vi "Handle Error.vi"(7 "Stop on Unhandled Error (T)":bool=TRUE, 8 "error in":errorcluster, 11 "Measurement":refnum<class "Measurement.lvclass">) -> (0 "handling error":errorcluster, 2 "Unhandled error":errorcluster, 3 "Measurement out":refnum<class "Measurement.lvclass">)   [LabVIEW 2019, in "Measurement.lvclass"]
doc: "JKI State Machine Objects (SMO) 1.0.0.11\nJKI - JKI\nCopyright (c) 2016, JKIJKI State Machine Objects (SMO) 1.3.0.56\nJKI - JKI\nCopyright (c) 2017, JKI"
uses:
  Measurement.lvclass
  <vilib>/JKI/JKI SMO/SMO/SMO.lvclass
panel:
  # "For instructions on how to use the JKI State Machine Objects, examples and video tutorials, visit:\nhttp://jki.net/state-machine-objects/\n\nJKI State Machine Objects™\nhttp://jki.net/state-machine-objects/\nCopyright (C) 2005-2015, JKI <info@jki.net>\nALL RIGHTS RESERVED"
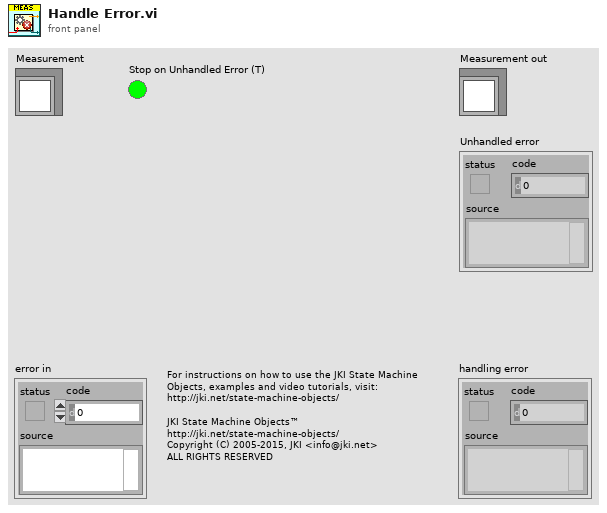
[diagram p1: front panel]
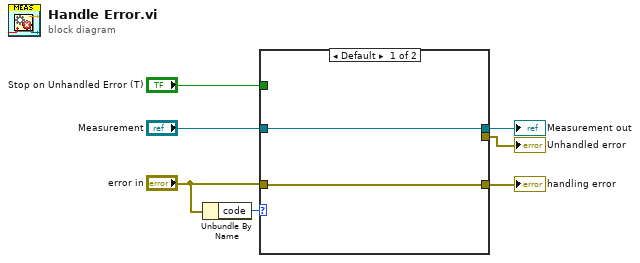
[diagram p0: block diagram]
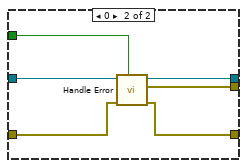
[diagram p2: hidden frame]
diagram:
  n1 = Unbundle By Name("error in") -> ("code"=w7:i32)
  n2 = case shown="Default" w7 {
    tunnel: "error in" -> [w8 w12]
    tunnel: "Measurement" -> [w9 w15]
    tunnel: [w9 w14] -> w4
    tunnel: "Stop on Unhandled Error (T)" -> [_ w13]
    tunnel: [w8 w11] -> w2
    tunnel: [_ w10] -> w1
    frame Default {
    }
    frame 0 {
      n3 = call-parent "Handle Error.vi"("Stop on Unhandled Error (T)"=w13, "error in"=w12, "SMO"=w15) -> ("handling error"=w11:errorcluster, "Unhandled error"=w10:errorcluster, "SMO out"=w14:refnum<class "Measurement.lvclass">)  [unwired: 6 in]
    }
  }
  "handling error" <- w2
  "Measurement out" <- w4
  "Unhandled error" <- w1
